vi "Sync Channel UI.vi"() -> ()   [LabVIEW 2025, in "Synchronization.lvlib" / "Synchronization Channel.lvclass"]
doc: "Copyright 2017 National Instruments Corporation\n\nLicensed under the Apache License, Version 2.0 (the \"License\"); you may not use this file except in compliance with the License. You may obtain a copy of the License at http://www.apache.org/licenses/LICENSE-2.0\nUnless required by applicable law or agreed to in writing, software distributed under the License is distributed on an \"AS IS\" BASIS, WITHOUT WARRANTIES OR CONDITIONS OF ANY KIND, either express or implied. See the License for the specific language governing permissions and limitations under the License."
uses:
  Synchronization Channel.lvclass
  Users/Public/Documents/Sandia National Labs/TSS Plugin/CEF.lvlibp/Node/NodeRef.ctl
  Users/Public/Documents/Sandia National Labs/TSS Plugin/CEF.lvlibp/Node/CEF_Node.lvclass
  Users/Public/Documents/Sandia National Labs/TSS Plugin/CEF.lvlibp/Node/mainQref.ctl
  Users/Public/Documents/Sandia National Labs/TSS Plugin/CEF.lvlibp/Node/UserEventRef.ctl
  Users/Public/Documents/Sandia National Labs/TSS Plugin/Abstract Engine.lvlibp/Plugin/Abstract/Channel configuration/Default Channel.ctl
  Synchronization Channel configuration/Sync Channel Setting.ctl
  Synchronization Channel.lvclass/Synchronization Channel.ctl
  Synchronization Channel configuration/Synchronization Channel configuration.lvclass/Synchronization Channel configuration.ctl
  Synchronization Channel configuration/Read Sync Channel Setting.vi
  Synchronization Channel configuration/Write Sync Channel Setting.vi
  <vilib>/Utility/error.llb/Trim Whitespace One-Sided.vi
  Synchronization Channel configuration/Synchronization Channel configuration.lvclass
  Users/Public/Documents/Sandia National Labs/TSS Plugin/Abstract Engine.lvlibp/Plugin/Abstract/Channel configuration/Read Channel Setting.vi
  Users/Public/Documents/Sandia National Labs/TSS Plugin/Abstract Engine.lvlibp/Plugin/Abstract/Channel configuration/Write Channel Setting.vi
  Users/Public/Documents/Sandia National Labs/TSS Plugin/Abstract Engine.lvlibp/Plugin/Abstract/Channel configuration/Channel configuration.lvclass
panel:
  in  "Sync Channel":cluster{"Default":T1, "Setting":T2}={"Default"={"Address"="None", "SW Alias"="None", "Enabled"=TRUE, "Type"="None", "Description"="* Type = Channel Class"}, "Setting"={"Inverter"=FALSE, "Update Edge"="Rising", "Source"="None", "Type"="None", "Synchronization Clock"="None", "Destination"="None"}}
  in  "user event":T3
  in  "main queue":T4
  in  "node ref":T5
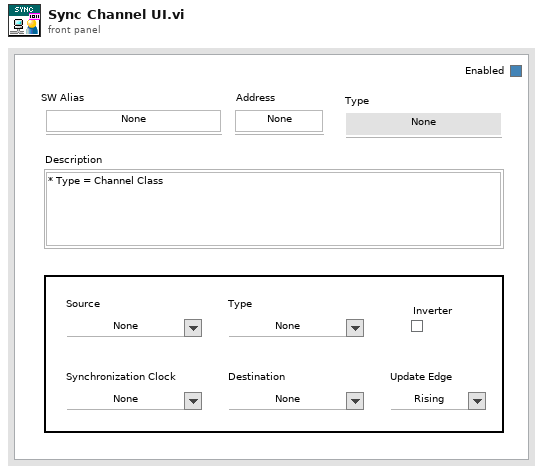
[diagram p1: front panel]
types:
  T1 = typedef "Abstract Engine.lvlibp/Channel configuration.lvclass/Default Channel.ctl" = cluster{"Address":string, "SW Alias":string, "Enabled":bool, "Type":string, "Description":string}
  T2 = typedef "Synchronization.lvlib/Synchronization Channel configuration.lvclass/Sync Channel Setting.ctl" = cluster{"Inverter":bool, "Update Edge":string, "Source":string, "Type":string, "Synchronization Clock":string, "Destination":string}
  T3 = typedef "CEF.lvlibp/CEF_Node.lvclass/UserEventRef.ctl" = refnum<user-event>
  T4 = typedef "CEF.lvlibp/CEF_Node.lvclass/mainQref.ctl" = refnum<queue>
  T5 = typedef "CEF.lvlibp/CEF_Node.lvclass/NodeRef.ctl" = refnum<data-value>
  T6 = cluster{"Channel Setting":T1, "Sync Channel Setting":T2}
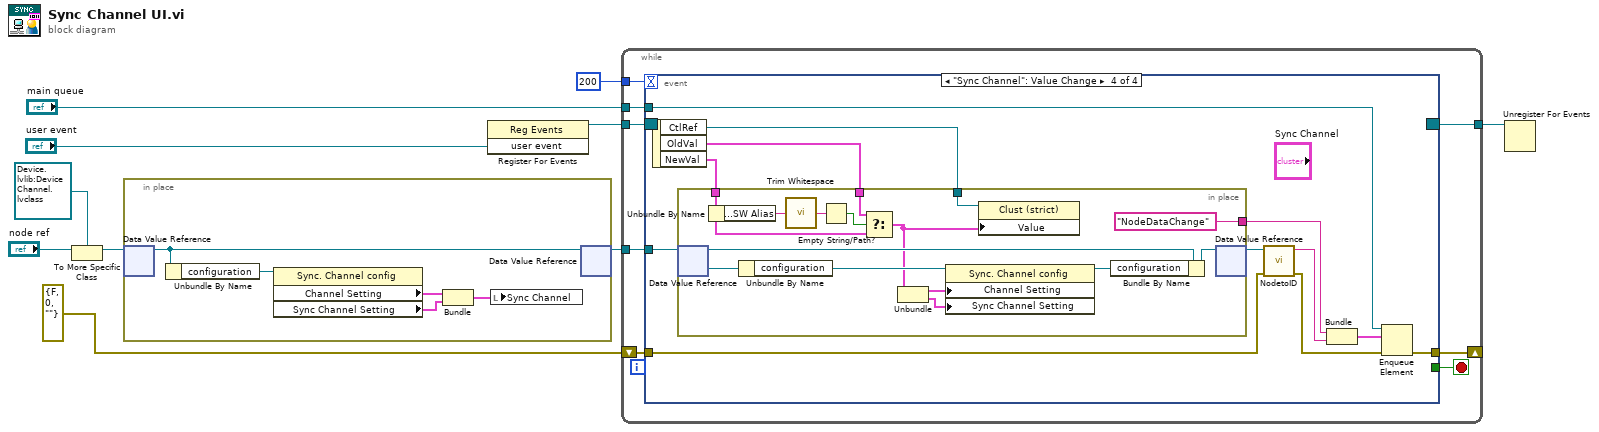
[diagram p0: block diagram]
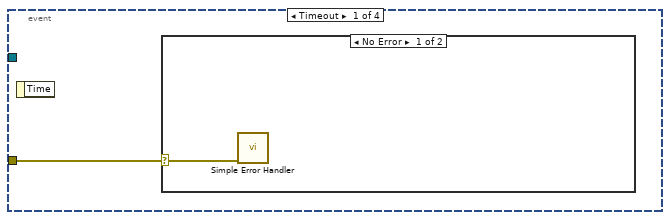
[diagram p2: hidden frame]
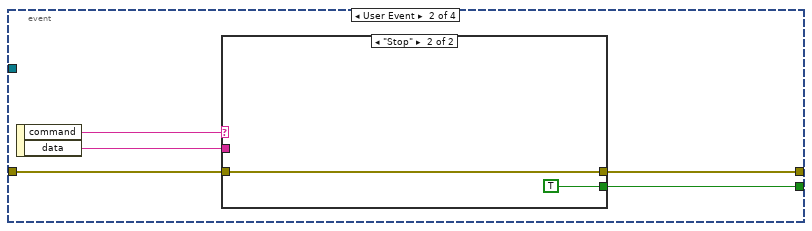
[diagram p4: hidden frame]
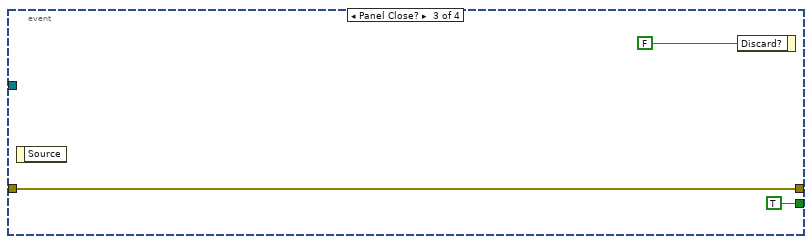
[diagram p6: hidden frame]
diagram:
  n1 = To More Specific Class(target class=refnum<data-value> refnum ("data value reference"), reference="node ref") -> (specific class reference=w6:refnum<data-value>)  [unwired: 1 in, 1 out]
  n2 = in-place {
    # "Initialize the front panel controls when loaded"
    n3 = in-place-dvr #1(w6) -> (w15:refnum<class "Synchronization Channel.lvclass">)  [unwired: 1 out]
    n4 = Unbundle By Name(w15) -> ("configuration"=w14:refnum<class "Synchronization Channel configuration.lvclass">)
    n5 = property class="Sync. Channel config"(reference=w14) -> ("Channel Setting"=w13:T1, "Sync Channel Setting"=w12:T2)  [unwired: 1 in, 2 out]
    n6 = Bundle("Channel Setting"=w13, "Sync Channel Setting"=w12) -> (w11:T6)  [unwired: 1 in]
    n7 = local write "Sync Channel"(w11) -> ()
    n8 = in-place-dvr #1(w15) -> (w5:refnum<data-value>)  [unwired: 1 out]
  }
  n9 = register-events("user event") -> (reference out=w9:refnum<event-registration>)  [unwired: 2 in, 1 out]
  n10 = while {
    tunnel: w5 -> [w23]
    tunnel: w9 -> [w22]
    tunnel: [w21] -> w8
    tunnel: "main queue" -> [w17]
    tunnel: 200 -> [w16]
    shift-right: [w18] -> _
    shift-left: errorcluster {"status"=FALSE, "code"=0, "source"=""} ("error out") -> [w19]
    stop <- w20 stop-if-true
    n11 = event shown="[3] \"Sync Channel\": Value Change" {
      selector: w22 -> [_ _ _ _]
      dyn-events: [_ _ _ _] -> w21
      timeout: w16 -> [_ _ _ _]
      tunnel: w23 -> [_ _ _ w46]
      tunnel: [_ w26 TRUE _] -> w20
      tunnel: [_ w27 w34 w47] -> w18
      tunnel: w19 -> [w24 w29 w34 w38]
      tunnel: w17 -> [_ _ _ w48]
      event Timeout {
        n12 = event-data() -> ()  [unwired: 1 in, 1 out]
        n13 = case shown="No Error" w24 {
          selector: w24 -> [w25 _]
          frame No Error {
            n14 = call <vilib>:"Simple Error Handler.vi"("error in (no error)"=w25) -> ()  [unwired: 4 in, 5 out]
          }
          frame Error {
          }
        }
      }
      event User Event {
        n15 = event-data() -> ("command"=w28:string, "data"=w30:string)  [unwired: 1 in]
        n16 = case shown="\"Stop\"" w28 {
          tunnel: [_ TRUE] -> w26
          tunnel: w30 -> [_ _]
          tunnel: w29 -> [w31 w32]
          tunnel: [w31 w32] -> w27
          frame Default {
          }
          frame "Stop" {
          }
        }
      }
      event Panel Close? {
        n17 = event-data() -> ()  [unwired: 1 in, 1 out]
        n18 = event-data("Discard?"=FALSE) -> ()  [unwired: 1 in, 1 out]
      }
      event "Sync Channel": Value Change {
        n19 = event-data() -> ("CtlRef"=w42:refnum<vi>, "OldVal"=w43:cluster{"Default":T1, "Setting":T2}, "NewVal"=w44:cluster{"Default":T1, "Setting":T2})  [unwired: 1 in]
        n20 = in-place {
          in-place-border: w44 -> [w55]
          in-place-border: w43 -> [w58]
          in-place-border: w42 -> [w57]
          in-place-border: ["NodeDataChange" ("Message Name")] -> w41
          n21 = in-place-dvr #2(w46) -> (w62:refnum<class "Synchronization Channel.lvclass">)  [unwired: 1 out]
          n22 = Unbundle By Name(w55) -> ("Default.SW Alias"=w56:string)
          n23 = Unbundle By Name(w62) -> ("configuration"=w61:refnum<class "Synchronization Channel configuration.lvclass">)
          n24 = call <vilib>:"Trim Whitespace.vi"("string"=w56) -> ("trimmed string"=w53:string)  [unwired: 1 in]
          n25 = Empty String/Path?(string/path=w53) -> (empty?=w54:bool)
          n26 = Select(t=w58, s=w54, f=w55) -> (s? t:f=w52:cluster{"Default":T1, "Setting":T2})
          n27 = Unbundle(w52) -> ("Default"=w49:T1, "Setting"=w51:T2)
          n28 = property class="Sync. Channel config"(reference=w61, "Channel Setting"=w49, "Sync Channel Setting"=w51) -> (reference out=w59:refnum<class "Synchronization Channel configuration.lvclass">)  [unwired: 1 in, 1 out]
          n29 = property class="Clust (strict)"(reference=w57, "Value"=w52) -> ()  [unwired: 1 in, 2 out]
          n30 = Bundle By Name(cluster=w62, "configuration"=w59) -> (w60:refnum<class "Synchronization Channel.lvclass">)
          n31 = in-place-dvr #2(w60) -> (w45:refnum<data-value>)  [unwired: 1 out]
        }
        n32 = call "NodetoID.vi"("error in"=w38, "node ref"=w45) -> ("error out"=w37:errorcluster, "ID"=w40:string)  [unwired: 8 in]
        n33 = Bundle("Message Name"=w41, "ID"=w40) -> (w39:cluster{"Message Name":string, "ID":string})  [unwired: 1 in]
        n34 = Enqueue Element(queue=w48, element=w39, error in (no error)=w37) -> (error out=w47:errorcluster)  [unwired: 1 in, 2 out]
      }
    }
  }
  n35 = Unregister For Events(event registration refnum=w8) -> ()  [unwired: 1 in, 1 out]
